vi "Append Point For Graph SubVi.vi"(1 "Numeric":dbl, 2 "Enum":T1, 3 "array":cluster{"X Cordinate":dbl, "Y Cordinate":dbl}[](array[cluster])) -> (0 "output array":cluster{"X Cordinate":dbl, "Y Cordinate":dbl}[](array[cluster]))   [LabVIEW 2017]
uses:
  Show Graph Inner Enum.ctl
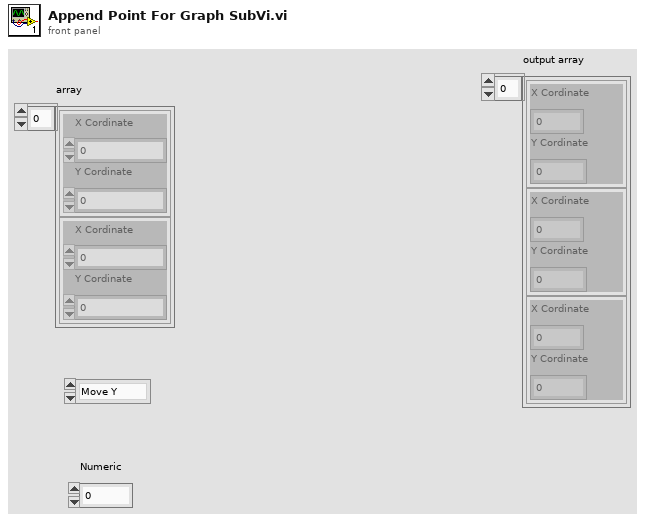
[diagram p1: front panel]
types:
  T1 = typedef "Show Graph Inner Enum.ctl" = enum16{"Move Y", "Move X", "Stop Command"}
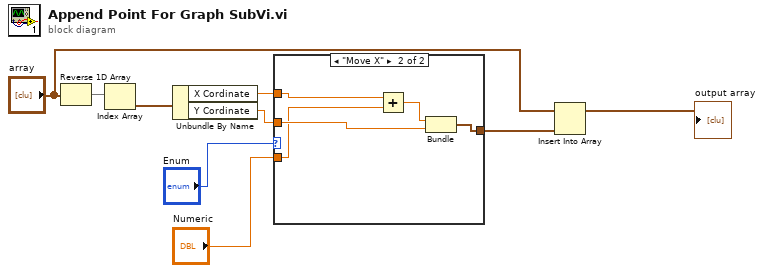
[diagram p0: block diagram]
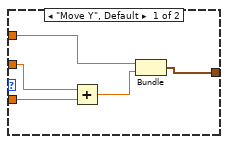
[diagram p2: hidden frame]
diagram:
  n1 = Reverse 1D Array(array="array") -> (reversed array=w8:cluster{"X Cordinate":dbl, "Y Cordinate":dbl}[])
  n2 = Index Array(array=w8) -> (element=w7:cluster{"X Cordinate":dbl, "Y Cordinate":dbl})  [unwired: 1 in]
  n3 = Unbundle By Name(w7) -> ("X Cordinate"=w6:dbl, "Y Cordinate"=w5:dbl)
  n4 = case shown="\"Move X\"" "Enum" {
    tunnel: w6 -> [w14 w17]
    tunnel: w5 -> [w13 w19]
    tunnel: "Numeric" -> [w12 w18]
    tunnel: [w10 w15] -> w2
    frame "Move Y", Default {
      n5 = Add(x=w13, y=w12) -> (x+y=w11:dbl)
      n6 = Bundle("X Cordinate"=w14, w11) -> (w10:cluster{"X Cordinate":dbl, dbl})  [unwired: 1 in]
    }
    frame "Move X" {
      n7 = Add(x=w17, y=w18) -> (x+y=w16:dbl)
      n8 = Bundle(w16, "Y Cordinate"=w19) -> (w15:cluster{dbl, "Y Cordinate":dbl})  [unwired: 1 in]
    }
  }
  n9 = Insert Into Array(array="array", new element=w2) -> (→"output array":cluster{"X Cordinate":dbl, "Y Cordinate":dbl}[])  [unwired: 1 in]
